vi "Sequencer Main.vi"() -> ()   [LabVIEW 2018] (continued)
                          n1247 = Unbundle By Name(w2009) -> ("Parameters"=w2004:string, "Step Description"=w2006:string)
                          n1248 = property on="Tab Control Msg" class="TabCtl (strict)"("Value"=T21."PowSupply" ("Tab Control Msg")) -> (error out=w2003:errorcluster)  [unwired: 2 in, 1 out]
                          n1249 = property on="Msg Str" class="Str"("Value"=w2006) -> ()  [unwired: 2 in, 2 out]
                          n1250 = in-place {
                            in-place-border: w2004 -> [w2027]
                            in-place-border: w2003 -> [_]
                            n1251 = while {
                              shift-right: [w2041] -> _
                              shift-left: w2027 -> [w2042]
                              tunnel: [w2038] -> w2034 mode=indexing
                              stop <- w2040 stop-if-true
                              # "Get Array of Parametrs"
                              n1252 = Match Pattern(string=w2042, regular expression=">") -> (before substring=w2038:string, after substring=w2041:string, offset past match=w2039:i32)  [unwired: 1 in, 1 out]
                              n1253 = Less Than 0?(x=w2039) -> (x < 0?=w2040:bool)
                            }
                            n1254 = global read "Global Variable.vi" "VISA Resource Name BK-9202"() -> (w2021:string)
                            n1255 = Index Array(array=w2034, index #1=0 ("index"), index #2=1 ("index"), index #3=2 ("index")) -> (element #1=w2026:string, element #2=w2023:string, element #3=w2014:string)
                            n1256 = To Upper Case(1:w2014) -> (0:w2013:string)
                            n1257 = Match Pattern(string=w2013, regular expression="ON") -> (offset past match=w2035:i32)  [unwired: 1 in, 3 out]
                            n1258 = Greater Than 0?(x=w2035) -> (x > 0?=w2019:bool)
                            n1259 = case shown="False" w2019 {
                              tunnel: [FALSE TRUE] -> w2010
                              frame False {
                              }
                              frame True {
                              }
                            }
                            n1260 = Scan From String(format string="%f", input string=w2026) -> (output 1=w2016:dbl)  [unwired: 3 in, 3 out]
                            n1261 = Scan From String(format string="%f", input string=w2023) -> (output 1=w2015:dbl)  [unwired: 3 in, 3 out]
                            n1262 = local read "PowSupply - SET"() -> (w2018:T7)
                            n1263 = call "bk9201 Set.vi"("Enable Output"=w2010, "Current"=w2015, "Voltage"=w2016, "VISA resource name"=w2021) -> ("error out"=w2020:errorcluster)  [unwired: 7 in]
                            n1264 = Bundle By Name(cluster=w2018, "ON/OFF"=w2010, "Volt (V)"=w2016, "Current Limit (A)"=w2015) -> (w2017:T7)
                            n1265 = global write "Global Variable.vi" "PowSupply ON/OFF"(w2010) -> ()
                            n1266 = global read "Global Variable.vi" "Array Errors"() -> (w2022:errorcluster[])
                            n1267 = local write "PowSupply - SET"(w2017) -> ()
                            n1268 = local read "Switch Relay Modules"() -> (w2012:T5)
                            n1269 = Bundle By Name(cluster=w2012, "Main Power Supplay ON/OFF"=w2010) -> (w2011:T5)
                            n1270 = Replace Array Subset(array=w2022, new element=w2020, index=2) -> (w2033:errorcluster[])
                            n1271 = global write "Global Variable.vi" "Array Errors"(w2033) -> ()
                            n1272 = local write "Switch Relay Modules"(w2011) -> ()
                          }
                          n1273 = case shown="True" FALSE {
                            frame False {
                            }
                            frame True {
                              n1274 = Wait (ms)(milliseconds to wait=u32 250) -> ()  [unwired: 1 out]
                            }
                          }
                        }
                        frame 16 {
                          # "PS Get Case"
                          # "Power Supplay - Get"
                          n1275 = Unbundle By Name(w2046) -> ("Parameters"=w2053:string, "Step Description"=w2052:string, "Test Values.Upper Limit"=w2051:dbl, "Test Values.Lower Limit"=w2050:dbl)
                          n1276 = property on="Tab Control Msg" class="TabCtl (strict)"("Value"=T21."PowSupply" ("Tab Control Msg")) -> (error out=w2047:errorcluster)  [unwired: 2 in, 1 out]
                          n1277 = property on="Msg Str" class="Str"("Value"=w2052) -> ()  [unwired: 2 in, 2 out]
                          n1278 = while {
                            shift-right: [w2061] -> _
                            shift-left: w2053 -> [w2062]
                            tunnel: w2051 -> [w2057]
                            tunnel: w2050 -> [w2056]
                            tunnel: [w2055] -> w2048
                            tunnel: [w2054] -> w2045
                            tunnel: w2047 -> [_]
                            stop <- w2060 stop-if-true
                            # "Lower Limit"
                            # "Upper Limit"
                            # "Get Array of Parametrs"
                            n1279 = Match Pattern(string=w2062, regular expression=";") -> (before substring=w2058:string, after substring=w2061:string, offset past match=w2059:i32)  [unwired: 1 in, 1 out]
                            n1280 = Less Or Equal To 0?(x=w2059) -> (x <= 0?=w2060:bool)
                            n1281 = in-place {
                              in-place-border: w2058 -> [w2080]
                              in-place-border: w2057 -> [w2070]
                              in-place-border: w2056 -> [w2069]
                              in-place-border: [w2073] -> w2055
                              in-place-border: [w2065] -> w2054
                              # "convert to mA"
                              n1282 = while {
                                shift-right: [w2113] -> _
                                shift-left: w2080 -> [w2114]
                                tunnel: [w2110] -> w2086 mode=indexing
                                stop <- w2112 stop-if-true
                                # "Get Array of Parametrs"
                                n1283 = Match Pattern(string=w2114, regular expression=">") -> (before substring=w2110:string, after substring=w2113:string, offset past match=w2111:i32)  [unwired: 1 in, 1 out]
                                n1284 = Less Or Equal To 0?(x=w2111) -> (x <= 0?=w2112:bool)
                              }
                              n1285 = global read "Global Variable.vi" "VISA Resource Name BK-9202"() -> (w2078:string)
                              n1286 = Index Array(array=w2086, index #1=0 ("index"), index #2=1 ("index"), index #3=2 ("index")) -> (element #1=w2074:string)  [unwired: 2 out]
                              n1287 = call "bk9201 Read.vi"("VISA resource name"=w2078) -> ("error out"=w2077:errorcluster, "Actual Power"=w2071:dbl, "Actual Current"=w2068:dbl, "Actual Voltage"=w2072:dbl)  [unwired: 7 in]
                              n1288 = Multiply(x=w2068, y=1000.0) -> (x*y=w2066:dbl)
                              n1289 = case shown="\"Volt?\"" w2074 {
                                tunnel: w2070 -> [_ w2093 w2100 w2107]
                                tunnel: w2069 -> [_ w2092 w2099 w2106]
                                tunnel: [enum16{"Idle", "PASS", "FALSE"}."Idle" ("Step Test Result") w2090 w2097 w2104] -> w2073
                                tunnel: w2066 -> [_ _ w2096 _]
                                tunnel: w2072 -> [_ w2089 _ _]
                                tunnel: w2071 -> [_ _ _ w2103]
                                frame "False", Default {
                                # "Step TEST Result"
                                n1290 = One Button Dialog(message="Ini File Err!") -> ()  [unwired: 1 in, 1 out]
                                }
                                frame "Volt?" {
                                n1291 = In Range and Coerce(upper limit=w2093, x=w2089, lower limit=w2092) -> (In Range?=w2091:bool)  [unwired: 1 out]
                                n1292 = case shown="True" w2091 {
                                tunnel: [enum16{"Idle", "PASS", "FALSE"}."FALSE" ("Step Test Result") enum16{"Idle", "PASS", "FALSE"}."PASS" ("Step Test Result")] -> w2090
                                frame False {
                                }
                                frame True {
                                # "Step TEST Result"
                                }
                                }
                                }
                                frame "Current?" {
                                n1293 = In Range and Coerce(upper limit=w2100, x=w2096, lower limit=w2099) -> (In Range?=w2098:bool)  [unwired: 1 out]
                                n1294 = case shown="False" w2098 {
                                tunnel: [enum16{"Idle", "PASS", "FALSE"}."FALSE" ("Step Test Result") enum16{"Idle", "PASS", "FALSE"}."PASS" ("Step Test Result")] -> w2097
                                frame False {
                                }
                                frame True {
                                # "Step TEST Result"
                                }
                                }
                                }
                                frame "Power?" {
                                n1295 = In Range and Coerce(upper limit=w2107, x=w2103, lower limit=w2106) -> (In Range?=w2105:bool)  [unwired: 1 out]
                                n1296 = case shown="False" w2105 {
                                tunnel: [enum16{"Idle", "PASS", "FALSE"}."FALSE" ("Step Test Result") enum16{"Idle", "PASS", "FALSE"}."PASS" ("Step Test Result")] -> w2104
                                frame False {
                                }
                                frame True {
                                # "Step TEST Result"
                                }
                                }
                                }
                              }
                              n1297 = local read "PowSupply - GET"() -> (w2076:T6)
                              n1298 = Bundle By Name(cluster=w2076, "Upper Limit"=w2070, "LowerLimit"=w2069, "Volt (V)"=w2072, "Current (mA)"=w2066, "Power (W)"=w2071) -> (w2075:T6)
                              n1299 = local write "PowSupply - GET"(w2075) -> ()
                              n1300 = global read "Global Variable.vi" "Array Errors"() -> (w2079:errorcluster[])
                              n1301 = Format Into String(format string="%.3f (mA)", w2066) -> (resulting string=w2065:string)  [unwired: 2 in, 1 out]
                              n1302 = Replace Array Subset(array=w2079, new element=w2077, index=2) -> (w2085:errorcluster[])
                              n1303 = global write "Global Variable.vi" "Array Errors"(w2085) -> ()
                            }
                          }
                        }
                        frame 20 {
                          # "Str \"fase\" Preset"
                          # "DMM Case"
                          # "DMM Case"
                          n1304 = in-place {
                            n1305 = local read "DMM Measure Monitor"() -> (w2175:T8)
                            n1306 = Bundle By Name(cluster=w2175, "Measure"="*****", "Mode"=T25."*****") -> (w2174:T8)
                            n1307 = local write "DMM Measure Monitor"(w2174) -> ()
                          }
                          n1308 = Unbundle By Name(w2131) -> ("Parameters"=w2122:string, "Test Values.Upper Limit"=w2127:dbl, "Test Values.Lower Limit"=w2125:dbl, "Test Values.Numeric Value"=w2126:dbl)
                          "Min" <- w2125
                          "Nominal" <- w2126
                          "Max" <- w2127
                          n1309 = in-place {
                            in-place-border: w2122 -> [w2145]
                            in-place-border: [w2141] -> w2121
                            in-place-border: [w2140] -> w2119
                            # "STr \"fase\" exist"
                            n1310 = To Lower Case(string=w2145) -> (all lower case string=w2146:string)
                            n1311 = Match Pattern(string=w2146, regular expression="false") -> (after substring=w2143:string, offset past match=w2142:i32)  [unwired: 1 in, 2 out]
                            n1312 = Greater Or Equal To 0?(x=w2142) -> (x >= 0?=w2140:bool)
                            n1313 = case shown="True" w2140 {
                              tunnel: w2143 -> [_ w2149]
                              tunnel: [string[] [] w2148] -> w2141
                              frame False {
                                (unwired) ""
                              }
                              frame True {
                                n1314 = while {
                                shift-right: [w2153] -> _
                                shift-left: w2149 -> [w2154]
                                tunnel: [w2150] -> w2148 mode=indexing
                                stop <- w2152 stop-if-true
                                # "Get Array of Sub Parametrs"
                                n1315 = Match Pattern(string=w2154, regular expression=":") -> (before substring=w2150:string, after substring=w2153:string, offset past match=w2151:i32)  [unwired: 1 in, 1 out]
                                n1316 = Less Than 0?(x=w2151) -> (x < 0?=w2152:bool)
                                }
                              }
                            }
                          }
                          n1317 = property on="Tab Control Msg" class="TabCtl (strict)"("Value"=T21."DMM" ("Tab Control Msg")) -> (error out=w2130:errorcluster)  [unwired: 2 in, 1 out]
                          n1318 = flat-sequence {
                            tunnel: w2126 -> [w2176]
                            tunnel: w2127 -> [w2179]
                            tunnel: w2125 -> [w2178]
                            tunnel: w2130 -> [_]
                            tunnel: [w2179] -> w2129
                            tunnel: [w2178] -> w2128
                            tunnel: w2129 -> [w2224]
                            tunnel: w2128 -> [w2223]
                            tunnel: [w2227] -> w2123
                            tunnel: w2122 -> [w2214]
                            tunnel: [w2215] -> w2124
                            frame #0 {
                              # "Lower Limit"
                              # "Upper Limit"
                              n1319 = Greater Than 0?(x=w2176) -> (x > 0?=w2177:bool)
                              n1320 = case shown="True" FALSE {
                                tunnel: w2179 -> [_ w2201]
                                tunnel: w2178 -> [_ w2200]
                                frame False {
                                }
                                frame True {
                                n1321 = Bundle By Name(cluster=T16 {"Step ID"=0, "Step Description"="", "Step Type"=0, "Test Values"={"Numeric Value"=0.0, "Str Value"="", "Boolean Value"=TRUE, "Upper Limit"=0.0, "Lower Limit"=0.0}, "Parameters"="", "Run/Skip"=TRUE, "Test Result"=enum."Idle", "Report"=TRUE, "Measure Units"="..."} ("Test Step"), "Test Values.Upper Limit"=w2201, "Test Values.Lower Limit"=w2200) -> (w2202:T16)
                                n1322 = global read "Global Variable.vi" "Current Step Nmb"() -> (w2204:u32)
                                n1323 = global read "Sequencer Array.vi" "SEQUENCER Array"() -> (w2206:T16[])
                                n1324 = Replace Array Subset(array=w2206, new element=w2202, index=w2204) -> (w2205:T16[])
                                n1325 = global write "Sequencer Array.vi" "SEQUENCER Array"(w2205) -> ()
                                }
                              }
                              n1326 = case shown="False" w2177 {
                                tunnel: [w2187 w2196] -> w2182
                                tunnel: [w2186 w2194] -> w2181
                                tunnel: w2179 -> [w2185 w2193]
                                tunnel: w2178 -> [w2184 w2192]
                                frame False {
                                n1327 = Multiply(x=w2184, y=0.2) -> (x*y=w2190:dbl)
                                n1328 = Multiply(x=w2185, y=-0.2) -> (x*y=w2191:dbl)
                                n1329 = Add(x=w2190, y=w2184) -> (x+y=w2186:dbl)
                                n1330 = Add(x=w2191, y=w2185) -> (x+y=w2187:dbl)
                                }
                                frame True {
                                n1331 = Multiply(x=w2192, y=-0.2) -> (x*y=w2195:dbl)
                                n1332 = Multiply(x=w2193, y=0.2) -> (x*y=w2197:dbl)
                                n1333 = Add(x=w2197, y=w2193) -> (x+y=w2196:dbl)
                                n1334 = Add(x=w2195, y=w2192) -> (x+y=w2194:dbl)
                                }
                              }
                              n1335 = Bundle("Lower Limit"=w2178, "Upper Limit"=w2179, "Numeric Value"=w2176) -> (w2183:T36)  [unwired: 1 in]
                              n1336 = property on="Limits" class="Slide (strict)"("Value"=w2183) -> ()  [unwired: 2 in, 2 out]
                              n1337 = property on="Limits" class="Slide (strict)"("Scale.Maximum"=w2182, "Scale.Minimum"=w2181) -> ()  [unwired: 2 in, 2 out]
                            }
                            frame #1 {
                              # "Element of Array the Data will be stored"
                              # "Open/Close"
                              n1338 = global read "Global Variable.vi" "VISA Resource Name BK-5492C"() -> (w2221:string)
                              n1339 = in-place {
                                (unwired) 11 items=["Voltage DC", "Voltage DC Ratio", "Voltage AC", "Current DC", "Current AC", "Resistance 2-Wire", "Resistance 4-Wire", "Frequency", "Period", "Capacitance", "Continuity", "Diode", "Temperature"] ("Measurement Function (0: Voltage DC)")
                              }
                              n1340 = Match Pattern(string=w2214, regular expression=">>") -> (after substring=w2209:string, offset past match=w2208:i32)  [unwired: 1 in, 2 out]
                              n1341 = call "BK-5492C_Main.vi"("Open/Close?"=TRUE, "Parameters"=w2214, "VISA resource name"=w2221) -> ("error out"=w2222:errorcluster, "Measurement Function"=w2220:i32, "Result Value"=w2216:dbl)  [unwired: 6 in]
                              n1342 = Greater Than 0?(x=w2208) -> (x > 0?=w2207:bool)
                              n1343 = case shown="11" w2220 {
                                tunnel: [T25."*****" ("Mode") T25."Voltage - DC" ("Mode") T25."Voltage - DC" ("Mode") T25."Voltage - AC" ("Mode") T25."Current - DC" ("Mode") T25."Current - AC" ("Mode") T25."Resistans 2-Wire" ("Mode") T25."Resistans 4-Wire" ("Mode") T25."*****" ("Mode") T25."*****" ("Mode") T25."Capasitor" ("Mode") T25."*****" ("Mode") T25."Diode" ("Mode")] -> w2219
                                tunnel: ["%.3f ***" ("format string") "%.3f (V)" "%.3f (V)" "%.3f (V)" "%.3f (A)" "%.3f (A)" w2253 w2276 "%.3f (HZ)" "%.3f ( ***)" ("format string") "%.3f (mF)" ("format string") "%.3f (***)" ("format string") "%.3f (V)" ("format string")] -> w2218
                                tunnel: w2216 -> [_ w2236 w2240 w2243 w2245 w2248 w2251 w2272 w2293 w2296 w2299 w2302 w2305]
                                tunnel: [0.0 ("Result Value") w2236 w2240 w2243 w2245 w2248 w2252 w2273 w2293 w2296 w2299 w2302 w2305] -> w2212
                                frame -1, Default {
                                }
                                frame 0 {
                                }
                                frame 1 {
                                }
                                frame 2 {
                                }
                                frame 3 {
                                }
                                frame 4 {
                                }
                                frame 5 {
                                # "Resistans 2-Wire"
                                n1344 = Greater?(x=w2251, y=1000.0) -> (0:w2255:bool)
                                n1345 = case shown="False" w2255 {
                                tunnel: ["%.3f (R)" w2259] -> w2253
                                tunnel: [w2257 w2263] -> w2252
                                tunnel: w2251 -> [w2257 w2262]
                                frame False {
                                }
                                frame True {
                                n1346 = Greater?(x=w2262, y=1000000.0) -> (0:w2260:bool)
                                n1347 = case shown="False" w2260 {
                                tunnel: [w2267 w2270] -> w2263
                                tunnel: w2262 -> [w2266 w2269]
                                tunnel: ["%.3f (K)" "%.3f (M)"] -> w2259
                                frame False {
                                n1348 = Divide(x=w2266, y=1000.0) -> (x/y=w2267:dbl)
                                }
                                frame True {
                                n1349 = Divide(x=w2269, y=1000000.0) -> (x/y=w2270:dbl)
                                }
                                }
                                }
                                }
                                }
                                frame 6 {
                                # "Resistans 4-Wire"
                                n1350 = Greater?(x=w2272, y=1000.0) -> (0:w2275:bool)
                                n1351 = case shown="False" w2275 {
                                tunnel: ["%.3f (R)" w2281] -> w2276
                                tunnel: w2272 -> [w2278 w2283]
                                tunnel: [w2278 w2280] -> w2273
                                frame False {
                                }
                                frame True {
                                n1352 = Greater?(x=w2283, y=1000000.0) -> (0:w2284:bool)
                                n1353 = case shown="False" w2284 {
                                tunnel: [w2288 w2291] -> w2280
                                tunnel: w2283 -> [w2287 w2290]
                                tunnel: ["%.3f (K)" "%.3f (M)"] -> w2281
                                frame False {
                                n1354 = Divide(x=w2287, y=1000.0) -> (x/y=w2288:dbl)
                                }
                                frame True {
                                n1355 = Divide(x=w2290, y=1000000.0) -> (x/y=w2291:dbl)
                                }
                                }
                                }
                                }
                                }
                                frame 7 {
                                }
                                frame 8 {
                                }
                                frame 9 {
                                }
                                frame 10 {
                                }
                                frame 11 {
                                }
                              }
                              n1356 = Decimal String To Number(string=w2209) -> (number=w2213:i32)  [unwired: 2 in, 1 out]
                              n1357 = local read "DMM Measure Monitor"() -> (w2226:T8)
                              n1358 = case shown="True" w2207 {
                                tunnel: w2213 -> [_ w2232]
                                tunnel: w2212 -> [_ w2231]
                                frame False {
                                }
                                frame True {
                                n1359 = global read "Global Variable.vi" "Array_Measurement"() -> (w2230:dbl[])
                                n1360 = Replace Array Subset(array=w2230, new element=w2231, index=w2232) -> (w2229:dbl[])
                                n1361 = global write "Global Variable.vi" "Array_Measurement"(w2229) -> ()
                                }
                              }
                              n1362 = Format Into String(format string=w2218, w2212) -> (resulting string=w2215:string)  [unwired: 2 in, 1 out]
                              n1363 = In Range and Coerce(upper limit=w2224, x=w2212, lower limit=w2223) -> (In Range?=w2228:bool)  [unwired: 1 out]
                              n1364 = in-place {
                                in-place-border: w2222 -> [w2308]
                                n1365 = global read "Global Variable.vi" "Array Errors"() -> (w2310:errorcluster[])
                                n1366 = Replace Array Subset(array=w2310, new element=w2308, index=1) -> (w2311:errorcluster[])
                                n1367 = global write "Global Variable.vi" "Array Errors"(w2311) -> ()
                              }
                              n1368 = Bundle("Lower Limit"=w2223, "Upper Limit"=w2224, "Result Value"=w2212) -> (w2211:T37)  [unwired: 1 in]
                              n1369 = property on="Limits" class="Slide (strict)"("Value"=w2211) -> ()  [unwired: 2 in, 2 out]
                              n1370 = Bundle By Name(cluster=w2226, "Measure"=w2215, "Mode"=w2219) -> (w2225:T8)
                              n1371 = case shown="False" w2228 {
                                tunnel: [enum16{"Idle", "PASS", "FALSE"}."FALSE" ("Step Test Result") enum16{"Idle", "PASS", "FALSE"}."PASS" ("Step Test Result")] -> w2227
                                frame False {
                                # "Step TEST Result"
                                }
                                frame True {
                                # "Step TEST Result"
                                }
                              }
                              n1372 = local write "DMM Measure Monitor"(w2225) -> ()
                            }
                          }
                          n1373 = local read "Debugging"() -> (w2120:bool)
                          n1374 = in-place {
                            in-place-border: w2121 -> [w2139]
                            in-place-border: [w2133] -> w2118
                            in-place-border: [w2132] -> w2117
                            # "GoTo Test-nmb"
                            # "ReTest Cyckles"
                            n1375 = Index Array(array=w2139, index #1=0, index #2=1, index #3=2) -> (element #2=w2135:string, element #3=w2134:string)  [unwired: 1 out]
                            n1376 = Decimal String To Number(string=w2135) -> (number=w2133:i32)  [unwired: 2 in, 1 out]
                            n1377 = Decimal String To Number(string=w2134) -> (number=w2132:i32)  [unwired: 2 in, 1 out]
                          }
                          n1378 = case shown="False" w2120 {
                            tunnel: w2119 -> [w2159 _]
                            tunnel: w2118 -> [w2157 _]
                            tunnel: w2117 -> [w2156 _]
                            frame False {
                              # "No Debug Mode"
                              n1379 = in-place {
                                in-place-border: [w2161] -> w2158
                                n1380 = global read "Global Variable.vi" "Retest Cnt"() -> (w2162:i16)
                                n1381 = Equal?(x=w2162, y=i16 0) -> (x = y?=w2161:bool)
                              }
                              n1382 = case shown="True" w2159 {
                                tunnel: w2158 -> [_ w2166]
                                tunnel: w2157 -> [_ w2164]
                                tunnel: w2156 -> [_ w2163]
                                frame False {
                                }
                                frame True {
                                # "String \"false\" Present"
                                n1383 = global write "Global Variable.vi" "Retest Step Nmb"(w2164) -> ()
                                n1384 = global write "Global Variable.vi" "Retest Nmb"(w2163) -> ()
                                n1385 = case shown="True" w2166 {
                                tunnel: w2163 -> [_ w2171]
                                frame False {
                                n1386 = global read "Global Variable.vi" "Retest Cnt"() -> (w2169:i16)
                                n1387 = Decrement(x=w2169) -> (x-1=w2168:i16)
                                n1388 = global write "Global Variable.vi" "Retest Cnt"(w2168) -> ()
                                n1389 = Wait (ms)(milliseconds to wait=u32 1000) -> ()  [unwired: 1 out]
                                }
                                frame True {
                                # "if(Retest-OFF & Cnt=0)"
                                n1390 = Decrement(x=w2171) -> (x-1=w2170:i32)
                                n1391 = global write "Global Variable.vi" "Retest Cnt"(w2170) -> ()
                                }
                                }
                                n1392 = global write "Global Variable.vi" "Retest ON"(TRUE ("Retest ON")) -> ()
                                }
                              }
                            }
                            frame True {
                            }
                          }
                        }
                        frame 40 {
                          # "U-Blox"
                          # "BlueTooht Case"
                          # "Test ADB Bluetooth"
                          n1393 = Unbundle By Name(w2328) -> ("Parameters"=w2319:string, "Step Description"=w2316:string, "Test Values.Upper Limit"=w2323:dbl, "Test Values.Lower Limit"=w2322:dbl)  [unwired: 1 out]
                          n1394 = in-place {
                            in-place-border: w2319 -> [w2443]
                            in-place-border: [w2439] -> w2318
                            in-place-border: [w2438] -> w2317
                            # "STr \"fase\" exist"
                            n1395 = To Lower Case(string=w2443) -> (all lower case string=w2444:string)
                            n1396 = Match Pattern(string=w2444, regular expression="false") -> (after substring=w2441:string, offset past match=w2440:i32)  [unwired: 1 in, 2 out]
                            n1397 = Greater Or Equal To 0?(x=w2440) -> (x >= 0?=w2438:bool)
                            n1398 = case shown="True" w2438 {
                              tunnel: w2441 -> [_ w2447]
                              tunnel: [string[] [] w2446] -> w2439
                              frame False {
                                (unwired) ""
                              }
                              frame True {
                                n1399 = while {
                                shift-right: [w2451] -> _
                                shift-left: w2447 -> [w2452]
                                tunnel: [w2448] -> w2446 mode=indexing
                                stop <- w2450 stop-if-true
                                # "Get Array of Sub Parametrs"
                                n1400 = Match Pattern(string=w2452, regular expression=":") -> (before substring=w2448:string, after substring=w2451:string, offset past match=w2449:i32)  [unwired: 1 in, 1 out]
                                n1401 = Less Than 0?(x=w2449) -> (x < 0?=w2450:bool)
                                }
                              }
                            }
                          }
                          n1402 = property on="Msg Str" class="Str"("Value"=w2316) -> ()  [unwired: 2 in, 2 out]
                          n1403 = property on="Tab Control Msg" class="TabCtl (strict)"("Value"=T4."Bluetooth" ("Tab Control Msg")) -> (error out=w2326:errorcluster)  [unwired: 2 in, 1 out]
                          n1404 = flat-sequence {
                            tunnel: w2326 -> [w2342]
                            tunnel: w2323 -> [w2340]
                            tunnel: w2322 -> [w2339]
                            tunnel: w2319 -> [w2335]
                            tunnel: [w2343] -> w2321
                            tunnel: [w2331] -> w2320
                            tunnel: w2316 -> [w2332]
                            tunnel: [w2330] -> w2315
                            tunnel: [w2329] -> w2314
                            tunnel: [w2402] -> w2324
                            tunnel: [w2408] -> w2327
                            tunnel: w2321 -> [w2408]
                            tunnel: w2320 -> [w2402]
                            tunnel: w2318 -> [w2407]
                            tunnel: w2317 -> [w2405]
                            tunnel: w2315 -> [w2401]
                            tunnel: w2314 -> [w2400]
                            frame #0 {
                              # "Step TEST Result"
                              n1405 = in-place {
                                in-place-border: w2335 -> [w2363]
                                in-place-border: w2342 -> [_]
                                in-place-border: [w2366] -> w2338
                                in-place-border: [w2365] -> w2336
                                in-place-border: [w2364] -> w2341
                                in-place-border: w2332 -> [w2361]
                                in-place-border: [w2362] -> w2330
                                in-place-border: [w2361] -> w2329
                                # "ADB BLE Name"
                                n1406 = in-place {
                                in-place-border: [w2388] -> w2366
                                in-place-border: [w2381] -> w2365
                                in-place-border: [w2380] -> w2364
                                in-place-border: [w2371] -> w2362
                                # "Bluetooth Test"
                                n1407 = vi-ref "ADB-BlueTooth.vi"() -> (w2372:refnum<vi>)
                                n1408 = property class="VI"(reference=w2372) -> (error out=w2377:errorcluster, "Path"=w2378:path)  [unwired: 1 in, 1 out]
                                n1409 = Open VI Reference(type specifier VI Refnum (for type only)=refnum<vi> refnum, vi path=w2378, error in (no error)=w2377) -> (vi reference=w2375:refnum<vi>, error out=w2374:errorcluster)  [unwired: 3 in]
                                n1410 = global read "Global Variable.vi" "COM Port BLE"() -> (w2379:refnum<visa-resource-name>)
                                n1411 = invoke on="Sub Panel" class="SubPnl" method="Insert VI"(error in=w2374, "VI Ref"=w2375) -> (error out=w2373:errorcluster)  [unwired: 2 in, 3 out]
                                n1412 = call-by-ref "?"(reference=w2375, error in=w2373, "COM Port"=w2379) -> (reference out=w2393:refnum<vi>, error out=w2392:errorcluster, 0:"error out"=w2385:errorcluster, "Connectet"=w2388:bool, "ADB PID"=w2384:string, "RSSI"=w2380:i32, "ADB Data Monitor"=w2371:string)  [unwired: 5 in, 1 out]
                                n1413 = global read "Global Variable.vi" "Array Errors"() -> (w2390:errorcluster[])
                                n1414 = Close Reference(reference=w2393, error in (no error)=w2392) -> (error out=w2387:errorcluster)
                                n1415 = Merge Errors(w2387, w2385) -> (w2386:errorcluster)
                                n1416 = String Subset(string=w2384, offset (0)=1, length (rest)=13 ("length (rest)")) -> (substring=w2381:string)
                                n1417 = Replace Array Subset(array=w2390, new element=w2386, index=15) -> (w2391:errorcluster[])
                                n1418 = global write "Global Variable.vi" "Array Errors"(w2391) -> ()
                                }
                                n1419 = while {
                                shift-right: [w2397] -> _
                                shift-left: w2363 -> [w2398]
                                tunnel: [w2394] -> w2367 mode=indexing
                                stop <- w2396 stop-if-true
                                # "Get Array of Parametrs"
                                n1420 = Match Pattern(string=w2398, regular expression=">") -> (before substring=w2394:string, after substring=w2397:string, offset past match=w2395:i32)  [unwired: 1 in, 1 out]
                                n1421 = Less Than 0?(x=w2395) -> (x < 0?=w2396:bool)
                                }
                                n1422 = Index Array(array=w2367, index #1=0 ("index"), index #2=1 ("index"), index #3=2 ("index")) -> ()  [unwired: 3 out]
                              }
                              n1423 = in-place {
                                in-place-border: [w2349] -> w2333
                                in-place-border: w2336 -> [w2348]
                                n1424 = global read "Global Variable.vi" "Rd PID"() -> (w2350:string)
                                n1425 = Equal?(x=w2350, y=w2348) -> (x = y?=w2349:bool)
                                n1426 = global write "Global Variable.vi" "Rd PID Ble"(w2348) -> ()
                              }
                              n1427 = in-place {
                                in-place-border: w2341 -> [w2345]
                                in-place-border: w2340 -> [w2347]
                                in-place-border: w2339 -> [w2346]
                                in-place-border: [w2344] -> w2337
                                n1428 = In Range and Coerce(upper limit=w2347, x=w2345, lower limit=w2346) -> (In Range?=w2344:bool)  [unwired: 1 out]
                              }
                              n1429 = case shown="True" w2333 {
                                tunnel: w2336 -> [_ w2352]
                                tunnel: ["BLE-PID (False)" w2358] -> w2331
                                tunnel: w2341 -> [_ w2357]
                                frame False {
                                }
                                frame True {
                                n1430 = Number To Decimal String(number=w2357) -> (decimal integer string=w2356:string)  [unwired: 1 in]
                                n1431 = Concatenate Strings(w2356, " (db) ", "\r\n", "BLE PID: ", w2352) -> (w2358:string)
                                }
                              }
                              n1432 = Compound Arithmetic op=AND(w2338, w2337, w2333) -> (w2334:bool)
                              n1433 = case shown="True" w2334 {
                                tunnel: [enum16{"Idle", "PASS", "FALSE"}."FALSE" ("Step Test Result") enum16{"Idle", "PASS", "FALSE"}."PASS" ("Step Test Result")] -> w2343
                                frame False {
                                }
                                frame True {
                                }
                              }
                            }
                            frame #1 {
                              # "Str \"fase\" Preset"
                              n1434 = in-place {
                                in-place-border: w2400 -> [w2411]
                                in-place-border: w2401 -> [w2410]
                                in-place-border: w2402 -> [w2409]
                                n1435 = call "Log Add Msg.vi"("Result"=w2409, "Communication"=w2410, "Description"=w2411) -> ("Out Msg"=w2412:string)
                                n1436 = property on="LogMsg" class="Str"("Text.Scroll Position"=inf) -> ()  [unwired: 2 in, 2 out]
                                n1437 = invoke on="LogMsg" class="Str" method="Append String"("string"=w2412) -> ()  [unwired: 3 in, 4 out]
                              }
                              n1438 = in-place {
                                in-place-border: w2407 -> [w2437]
                                in-place-border: [w2431] -> w2404
                                in-place-border: [w2430] -> w2403
                                # "GoTo Test-nmb"
                                # "ReTest Cyckles"
                                n1439 = Index Array(array=w2437, index #1=0, index #2=1, index #3=2) -> (element #2=w2433:string, element #3=w2432:string)  [unwired: 1 out]
                                n1440 = Decimal String To Number(string=w2433) -> (number=w2431:i32)  [unwired: 2 in, 1 out]
                                n1441 = Decimal String To Number(string=w2432) -> (number=w2430:i32)  [unwired: 2 in, 1 out]
                              }
                              n1442 = local read "Debugging"() -> (w2406:bool)
                              n1443 = case shown="False" w2406 {
                                tunnel: w2405 -> [w2417 _]
                                tunnel: w2404 -> [w2415 _]
                                tunnel: w2403 -> [w2414 _]
                                frame False {
                                # "No Debug Mode"
                                n1444 = in-place {
                                in-place-border: [w2419] -> w2416
                                n1445 = global read "Global Variable.vi" "Retest Cnt"() -> (w2420:i16)
                                n1446 = Equal?(x=w2420, y=i16 0) -> (x = y?=w2419:bool)
                                }
                                n1447 = case shown="True" w2417 {
                                tunnel: w2416 -> [_ w2424]
                                tunnel: w2415 -> [_ w2422]
                                tunnel: w2414 -> [_ w2421]
                                frame False {
                                }
                                frame True {
                                # "String \"false\" Present"
                                n1448 = global write "Global Variable.vi" "Retest Step Nmb"(w2422) -> ()
                                n1449 = global write "Global Variable.vi" "Retest Nmb"(w2421) -> ()
                                n1450 = case shown="False" w2424 {
                                tunnel: w2421 -> [_ w2429]
                                frame False {
                                n1451 = global read "Global Variable.vi" "Retest Cnt"() -> (w2427:i16)
                                n1452 = Decrement(x=w2427) -> (x-1=w2426:i16)
                                n1453 = global write "Global Variable.vi" "Retest Cnt"(w2426) -> ()
                                n1454 = Wait (ms)(milliseconds to wait=u32 1000) -> ()  [unwired: 1 out]
                                }
                                frame True {
                                # "if(Retest-OFF & Cnt=0)"
                                n1455 = Decrement(x=w2429) -> (x-1=w2428:i32)
                                n1456 = global write "Global Variable.vi" "Retest Cnt"(w2428) -> ()
                                }
                                }
                                n1457 = global write "Global Variable.vi" "Retest ON"(TRUE ("Retest ON")) -> ()
                                }
                                }
                                }
                                frame True {
                                }
                              }
                            }
                          }
                        }
                        frame 41 {
                          # "Esp-32"
                          # "BlueTooht Case"
                          # "Test ADB Bluetooth"
                          n1458 = Unbundle By Name(w2470) -> ("Parameters"=w2461:string, "Step Description"=w2458:string, "Test Values.Upper Limit"=w2465:dbl, "Test Values.Lower Limit"=w2464:dbl)  [unwired: 1 out]
                          n1459 = in-place {
                            in-place-border: w2461 -> [w2576]
                            in-place-border: [w2572] -> w2460
                            in-place-border: [w2571] -> w2459
                            # "Str \"fase\" exist"
                            n1460 = To Lower Case(string=w2576) -> (all lower case string=w2577:string)
                            n1461 = Match Pattern(string=w2577, regular expression="false") -> (after substring=w2574:string, offset past match=w2573:i32)  [unwired: 1 in, 2 out]
                            n1462 = Greater Or Equal To 0?(x=w2573) -> (x >= 0?=w2571:bool)
                            n1463 = case shown="True" w2571 {
                              tunnel: w2574 -> [_ w2580]
                              tunnel: [string[] [] w2579] -> w2572
                              frame False {
                                (unwired) ""
                              }
                              frame True {
                                n1464 = while {
                                shift-right: [w2584] -> _
                                shift-left: w2580 -> [w2585]
                                tunnel: [w2581] -> w2579 mode=indexing
                                stop <- w2583 stop-if-true
                                # "Get Array of Sub Parametrs"
                                n1465 = Match Pattern(string=w2585, regular expression=":") -> (before substring=w2581:string, after substring=w2584:string, offset past match=w2582:i32)  [unwired: 1 in, 1 out]
                                n1466 = Less Than 0?(x=w2582) -> (x < 0?=w2583:bool)
                                }
                              }
                            }
                          }
                          n1467 = property on="Msg Str" class="Str"("Value"=w2458) -> ()  [unwired: 2 in, 2 out]
                          n1468 = global read "Global Variable.vi" "COM Port BLE"() -> (w2455:refnum<visa-resource-name>)
                          n1469 = invoke on="Serial CMD Mon" class="Str" method="Reinit To Default"() -> (error out=w2454:errorcluster)  [unwired: 3 in, 2 out]
                          n1470 = property on="Tab Control Msg" class="TabCtl (strict)"("Value"=T4."Serial" ("Tab Control Msg")) -> (error out=w2468:errorcluster)  [unwired: 2 in, 1 out]
                          n1471 = flat-sequence {
                            tunnel: w2468 -> [w2490]
                            tunnel: w2465 -> [w2489]
                            tunnel: w2464 -> [w2488]
                            tunnel: w2461 -> [w2487]
                            tunnel: [w2491] -> w2463
                            tunnel: [w2484] -> w2462
                            tunnel: w2458 -> [w2485]
                            tunnel: [w2483] -> w2457
                            tunnel: [w2482] -> w2456
                            tunnel: w2455 -> [w2481]
                            tunnel: w2454 -> [_]
                            tunnel: [w2535] -> w2466
                            tunnel: [w2541] -> w2469
                            tunnel: w2463 -> [w2541]
                            tunnel: w2462 -> [w2535]
                            tunnel: w2460 -> [w2540]
                            tunnel: w2459 -> [w2538]
                            tunnel: w2457 -> [w2534]
                            tunnel: w2456 -> [w2533]
                            frame #0 {
                              # "Step TEST Description"
                              # "Step TEST Result"
                              n1472 = in-place {
                                in-place-border: w2487 -> [w2510]
                                in-place-border: w2490 -> [_]
                                in-place-border: w2485 -> [w2509]
                                in-place-border: [w2503] -> w2483
                                in-place-border: [w2509] -> w2482
                                in-place-border: w2481 -> [w2508]
                                in-place-border: [w2506] -> w2480
                                in-place-border: [w2502] -> w2478
                                in-place-border: [w2505] -> w2477
                                in-place-border: [w2504] -> w2476
                                in-place-border: [w2504] -> w2475
                                # "ADB BLE Name"
                                n1473 = while {
                                shift-right: [w2530] -> _
                                shift-left: w2510 -> [w2531]
                                tunnel: [w2527] -> w2511 mode=indexing
                                stop <- w2529 stop-if-true
                                # "Get Array of Parametrs"
                                n1474 = Match Pattern(string=w2531, regular expression=">") -> (before substring=w2527:string, after substring=w2530:string, offset past match=w2528:i32)  [unwired: 1 in, 1 out]
                                n1475 = Less Than 0?(x=w2528) -> (x < 0?=w2529:bool)
                                }
                                n1476 = global read "Global Variable.vi" "Baccode MEM"() -> (w2501:string)
                                n1477 = control-ref of="Serial CMD Mon"() -> (w2507:refnum<vi>)
                                n1478 = Select(t=w2501, s=TRUE, f="2210070000001") -> (s? t:f=w2500:string)
                                n1479 = Index Array(array=w2511, index #1=0 ("index"), index #2=1 ("index"), index #3=2 ("index")) -> ()  [unwired: 3 out]
                                n1480 = call "ADB-LMS_Esp32.vi"("Monitor Refnum"=w2507, "Serial PID"=w2500, "COM BLE Esp32"=w2508) -> ("Check  BLE"=w2506:bool, "CMD Monitor"=w2503:string, "BLE PID Str"=w2505:string)  [unwired: 5 in, 1 out]
                                n1481 = case shown="True" w2506 {
                                tunnel: w2503 -> [_ w2526]
                                tunnel: [FALSE w2525] -> w2502
                                tunnel: [0 ("rssi") w2524] -> w2504
                                frame False {
                                }
                                frame True {
                                n1482 = local read "Barcode"() -> (w2523:string)
                                n1483 = call <vilib>:"Space Constant.vi"() -> ("String"=w2519:string)
                                n1484 = String Subset(string=w2523, offset (0)=0, length (rest)=13 ("length (rest)")) -> (substring=w2517:string)
                                n1485 = Concatenate Strings("LEDLMS" ("BLE Server Name"), w2519, w2517) -> (w2518:string)
                                n1486 = call "Get RSSI.vi"("BLE Server Name"=w2518, "CMD Monitor"=w2526) -> ("rssi"=w2524:i32, "BLE LMS Server Found"=w2525:bool)  [unwired: 7 in, 1 out]
                                }
                                }
                                n1487 = global write "Global Variable.vi" "Rd PID Ble"(w2505) -> ()
                              }
                              n1488 = in-place {
                                in-place-border: w2475 -> [w2493]
                                in-place-border: w2489 -> [w2495]
                                in-place-border: w2488 -> [w2494]
                                in-place-border: [w2492] -> w2479
                                n1489 = In Range and Coerce(upper limit=w2495, x=w2493, lower limit=w2494) -> (In Range?=w2492:bool)  [unwired: 1 out]
                              }
                              n1490 = Number To Decimal String(number=w2476) -> (decimal integer string=w2474:string)  [unwired: 1 in]
                              n1491 = Compound Arithmetic op=AND(w2479, w2478, w2480) -> (w2486:bool)
                              n1492 = Concatenate Strings(w2474, " (db) ", "\r\n", "BLE PID: ", w2477) -> (w2484:string)
                              n1493 = case shown="True" w2486 {
                                tunnel: [enum16{"Idle", "PASS", "FALSE"}."FALSE" ("Step Test Result") enum16{"Idle", "PASS", "FALSE"}."PASS" ("Step Test Result")] -> w2491
                                frame False {
                                }
                                frame True {
                                }
                              }
                            }
                            frame #1 {
                              # "Str \"fase\" Present"
                              n1494 = in-place {
                                in-place-border: w2533 -> [w2544]
                                in-place-border: w2534 -> [w2543]
                                in-place-border: w2535 -> [w2542]
                                n1495 = call "Log Add Msg.vi"("Result"=w2542, "Communication"=w2543, "Description"=w2544) -> ("Out Msg"=w2545:string)
                                n1496 = property on="LogMsg" class="Str"("Text.Scroll Position"=inf) -> ()  [unwired: 2 in, 2 out]
                                n1497 = invoke on="LogMsg" class="Str" method="Append String"("string"=w2545) -> ()  [unwired: 3 in, 4 out]
                              }
                              n1498 = in-place {
                                in-place-border: w2540 -> [w2570]
                                in-place-border: [w2564] -> w2537
                                in-place-border: [w2563] -> w2536
                                # "GoTo Test-nmb"
                                # "ReTest Cyckles"
                                n1499 = Index Array(array=w2570, index #1=0, index #2=1, index #3=2) -> (element #2=w2566:string, element #3=w2565:string)  [unwired: 1 out]
                                n1500 = Decimal String To Number(string=w2566) -> (number=w2564:i32)  [unwired: 2 in, 1 out]
                                n1501 = Decimal String To Number(string=w2565) -> (number=w2563:i32)  [unwired: 2 in, 1 out]
                              }
                              n1502 = local read "Debugging"() -> (w2539:bool)
                              n1503 = case shown="False" w2539 {
                                tunnel: w2538 -> [w2550 _]
                                tunnel: w2537 -> [w2548 _]
                                tunnel: w2536 -> [w2547 _]
                                frame False {
                                # "No Debug Mode"
                                n1504 = in-place {
                                in-place-border: [w2552] -> w2549
                                n1505 = global read "Global Variable.vi" "Retest Cnt"() -> (w2553:i16)
                                n1506 = Equal?(x=w2553, y=i16 0) -> (x = y?=w2552:bool)
                                }
                                n1507 = case shown="True" w2550 {
                                tunnel: w2549 -> [_ w2557]
                                tunnel: w2548 -> [_ w2555]
                                tunnel: w2547 -> [_ w2554]
                                frame False {
                                }
                                frame True {
                                # "String \"false\" Present"
                                n1508 = global write "Global Variable.vi" "Retest Step Nmb"(w2555) -> ()
                                n1509 = global write "Global Variable.vi" "Retest Nmb"(w2554) -> ()
                                n1510 = case shown="False" w2557 {
                                tunnel: w2554 -> [_ w2562]
                                frame False {
                                n1511 = global read "Global Variable.vi" "Retest Cnt"() -> (w2560:i16)
                                n1512 = Decrement(x=w2560) -> (x-1=w2559:i16)
                                n1513 = global write "Global Variable.vi" "Retest Cnt"(w2559) -> ()
                                n1514 = Wait (ms)(milliseconds to wait=u32 1000) -> ()  [unwired: 1 out]
                                }
                                frame True {
                                # "if(Retest-OFF & Cnt=0)"
                                n1515 = Decrement(x=w2562) -> (x-1=w2561:i32)
                                n1516 = global write "Global Variable.vi" "Retest Cnt"(w2561) -> ()
                                }
                                }
